vi "Add Interlock.vi"(6 "Add to (Deny)":T1, 8 "error in (no error)":errorcluster, 10 "Interlock.lvclass":refnum<class "Interlock.lvclass">, 11 "Interlock Chain in":refnum<class "Interlock Chain.lvclass">) -> (0 "error out":errorcluster, 3 "Interlock Chain out":refnum<class "Interlock Chain.lvclass">)   [LabVIEW 2015, in "Interlocks.lvlib" / "Interlock Chain.lvclass"]
uses:
  Interlock Chain.lvclass
  Interlock/Interlock.lvclass
  Controls/Add IL to -Enumerator.ctl
  Interlock Chain.lvclass/Interlock Chain.ctl
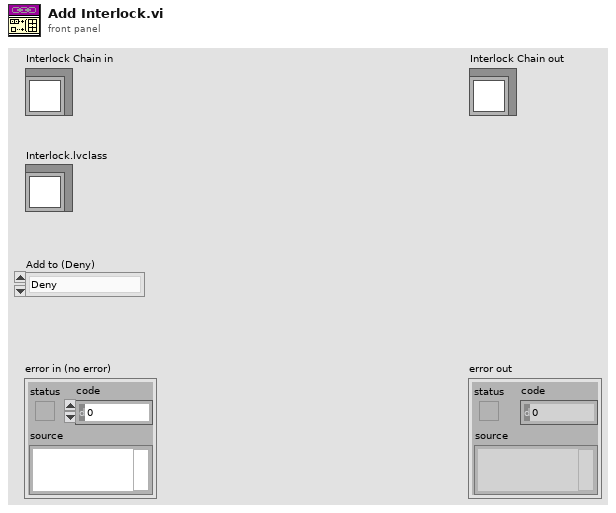
[diagram p1: front panel]
types:
  T1 = typedef "Add IL to -Enumerator.ctl" = enum16{"Deny", "Allow", "None"}
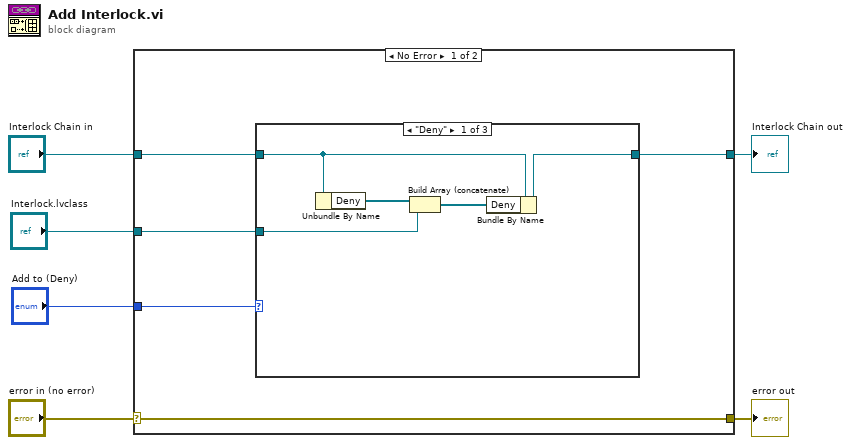
[diagram p0: block diagram]
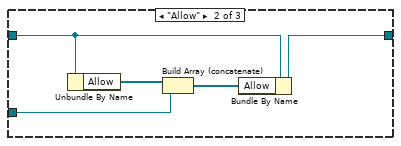
[diagram p2: hidden frame]
diagram:
  n1 = case shown="No Error" "error in (no error)" {
    selector: "error in (no error)" -> [w11 w24]
    tunnel: [w11 w24] -> w5
    tunnel: [w7 w23] -> w3
    tunnel: "Interlock Chain in" -> [w10 w23]
    tunnel: "Interlock.lvclass" -> [w8 _]
    tunnel: "Add to (Deny)" -> [w9 _]
    frame No Error {
      n2 = case shown="\"Deny\"" w9 {
        tunnel: w10 -> [w14 w19 w22]
        tunnel: w8 -> [w15 w20 _]
        tunnel: [w13 w18 w22] -> w7
        frame "Deny" {
          n3 = Unbundle By Name(w14) -> ("Deny"=w16:refnum<class "Interlock.lvclass">[])
          n4 = Build Array (concatenate)(w16, w15) -> (w12:refnum<class "Interlock.lvclass">[])
          n5 = Bundle By Name(cluster=w14, "Deny"=w12) -> (w13:refnum<class "Interlock Chain.lvclass">)
        }
        frame "Allow" {
          n6 = Unbundle By Name(w19) -> ("Allow"=w21:refnum<class "Interlock.lvclass">[])
          n7 = Build Array (concatenate)(w21, w20) -> (w17:refnum<class "Interlock.lvclass">[])
          n8 = Bundle By Name(cluster=w19, "Allow"=w17) -> (w18:refnum<class "Interlock Chain.lvclass">)
        }
        frame "None" {
        }
      }
    }
    frame Error {
    }
  }
  "error out" <- w5
  "Interlock Chain out" <- w3
